vi "Patch of Unflatten Json String.vi"(7 "VCluster":variant, 8 "error in (no error)":errorcluster, 11 "Variant in":variant) -> (0 "error out":errorcluster, 3 "Variant out":variant)   [LabVIEW 2019, in "lv-apt-json-file.lvlib"]
uses:
  lv-apt-json-file.lvlib
  <vilib>/Utility/Data Type/NI_Data Type.lvlib
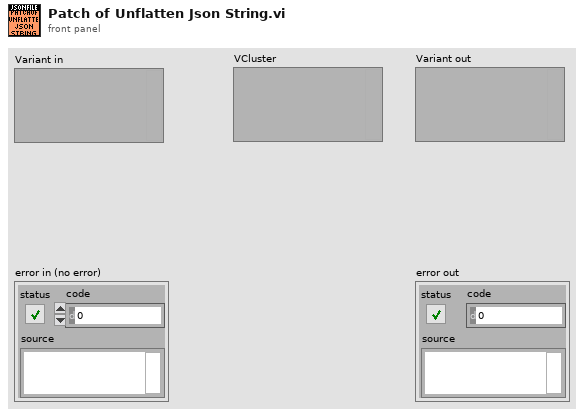
[diagram p1: front panel]
types:
  T1 = typedef "NI_Data Type.lvlib/Data Type.ctl" = enum8{"Invalid Type", "Void", "I8", "I16", "I32", "I64", "U8", "U16", "U32", "U64", "Single Float", "Double Float", "Extended Float", "Single Complex", "Double Complex", "Extended Complex", "Enum U8", "Enum U16", "Enum U32", "Enum U64", "Single Float With Unit", "Double Float With Unit", "Extended Float With Unit", "Single Complex with Unit", "Double Complex with Unit", "Extended Complex with Unit", "Boolean", "String", "Path", "Picture", "Tag", "Array", "Cluster", "Variant", "LV Variant", "Waveform", "Timestamp", "Digital Waveform", "Digital Data", "ExpressData", "Refnum", "External Data", "VI", "Poly VI", "LabVIEW Class Instance", "Fixed Point", "Set Collection", "Map Collection"}
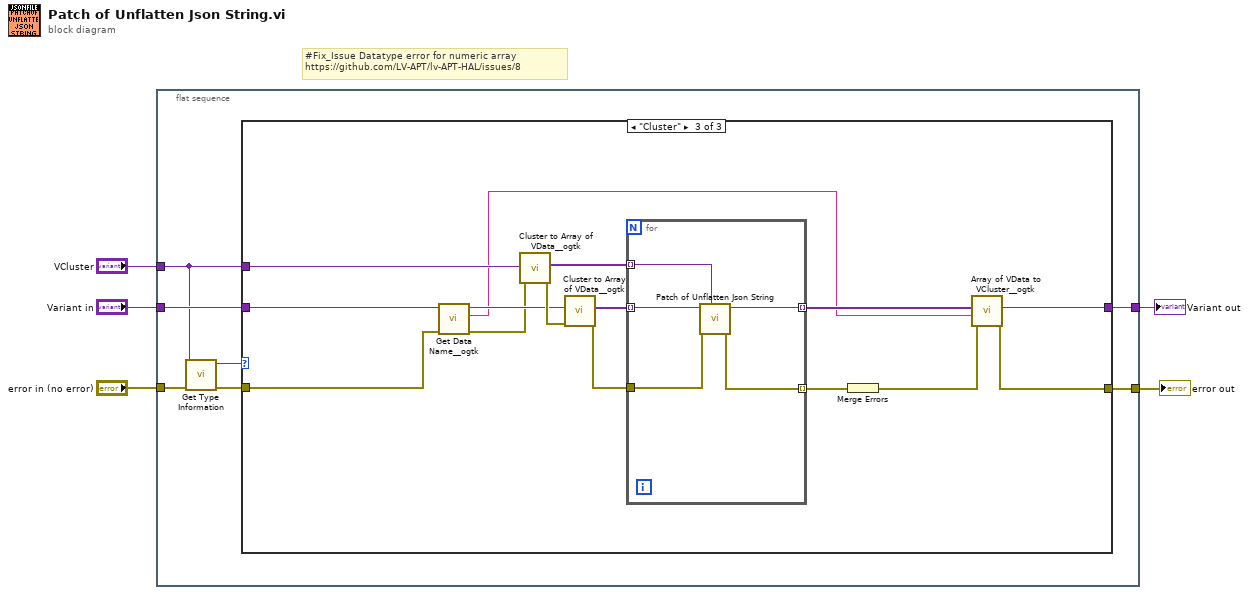
[diagram p0: block diagram]
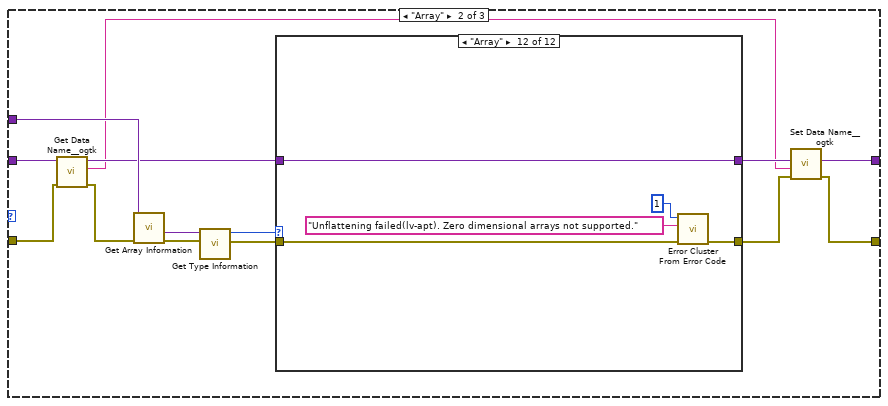
[diagram p3: hidden frame]
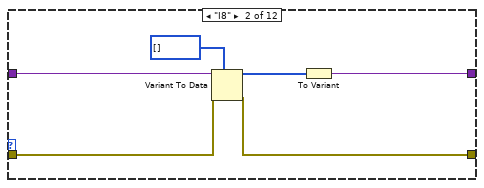
[diagram p5: hidden frame]
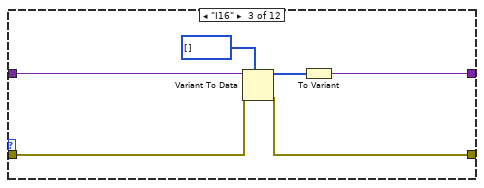
[diagram p6: hidden frame]
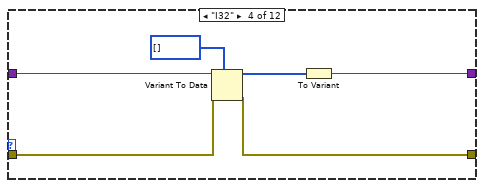
[diagram p7: hidden frame]
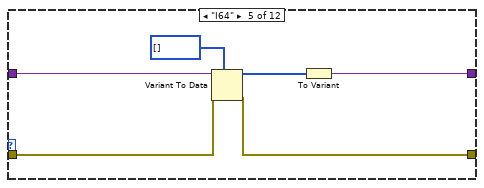
[diagram p8: hidden frame]
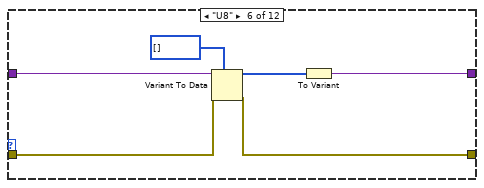
[diagram p9: hidden frame]
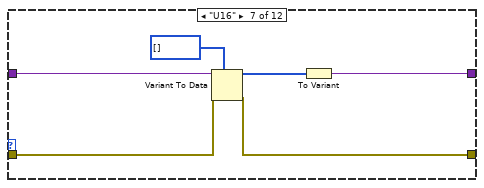
[diagram p10: hidden frame]
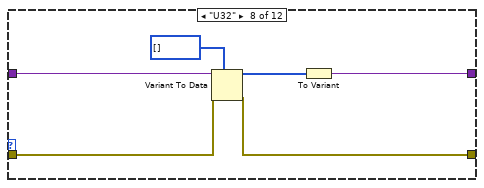
[diagram p11: hidden frame]
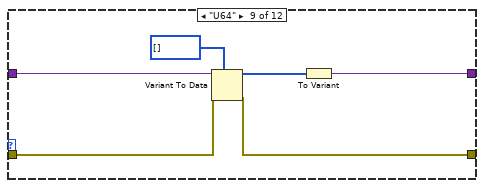
[diagram p12: hidden frame]
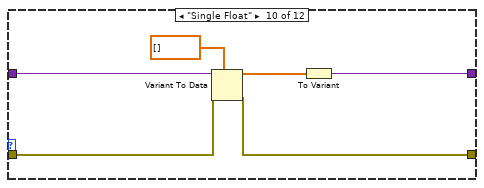
[diagram p13: hidden frame]
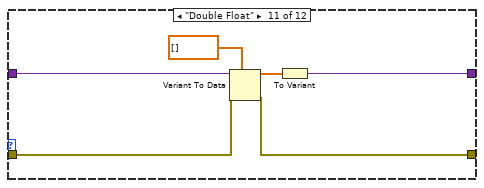
[diagram p14: hidden frame]
diagram:
  # "#Fix_Issue Datatype error for numeric array\nhttps://github.com/LV-APT/lv-APT-HAL/issues/8"
  n1 = flat-sequence {
    tunnel: [w12] -> w1
    tunnel: "Variant in" -> [w11]
    tunnel: "error in (no error)" -> [w9]
    tunnel: [w7] -> w4
    tunnel: "VCluster" -> [w6]
    frame #0 {
      n2 = call <vilib>:"Get Type Information.vi"("error in (no error)"=w9, "variant"=w6) -> ("error out"=w8:errorcluster, "type"=w10:T1)  [unwired: 5 in, 3 out]
      n3 = case shown="\"Cluster\"" w10 {
        tunnel: w11 -> [w14 w24 w110]
        tunnel: [w14 w20 w103] -> w12
        tunnel: w8 -> [w13 w19 w96]
        tunnel: [w13 w15 w100] -> w7
        tunnel: w6 -> [_ w22 w109]
        frame "Invalid Type", Default {
        }
        frame "Array" {
          n4 = call <userlib>:"Get Data Name__ogtk.vi"("error in (no error)"=w19, "Data"=w24) -> ("error out"=w18:errorcluster, "Data Name"=w17:string, "Data dup"=w21:variant)  [unwired: 7 in]
          n5 = call <vilib>:"Get Array Information.vi"("error in (no error)"=w18, "variant"=w22) -> ("error out"=w27:errorcluster, "array element data type"=w28:variant)  [unwired: 6 in, 2 out]
          n6 = call <vilib>:"Get Type Information.vi"("error in (no error)"=w27, "variant"=w28) -> ("error out"=w25:errorcluster, "type"=w26:T1)  [unwired: 5 in, 3 out]
          n7 = case shown="\"Array\"" w26 {
            tunnel: w25 -> [w29 w35 w41 w47 w53 w59 w65 w71 w77 w83 w89 w93]
            tunnel: [w29 w34 w40 w46 w52 w58 w64 w70 w76 w82 w88 w92] -> w16
            tunnel: w21 -> [w30 w36 w42 w48 w54 w60 w66 w72 w78 w84 w90 w91]
            tunnel: [w30 w31 w37 w43 w49 w55 w61 w67 w73 w79 w85 w91] -> w23
            frame Default {
            }
            frame "I8" {
              n8 = Variant To Data(error in=w35, type=i8[] [], Variant=w36) -> (data=w32:i8[], error out=w34:errorcluster)
              n9 = To Variant(anything=w32) -> (Variant=w31:variant)
            }
            frame "I16" {
              n10 = Variant To Data(error in=w41, type=i16[] [], Variant=w42) -> (data=w38:i16[], error out=w40:errorcluster)
              n11 = To Variant(anything=w38) -> (Variant=w37:variant)
            }
            frame "I32" {
              n12 = Variant To Data(error in=w47, type=i32[] [], Variant=w48) -> (data=w44:i32[], error out=w46:errorcluster)
              n13 = To Variant(anything=w44) -> (Variant=w43:variant)
            }
            frame "I64" {
              n14 = Variant To Data(error in=w53, type=i64[] [], Variant=w54) -> (data=w50:i64[], error out=w52:errorcluster)
              n15 = To Variant(anything=w50) -> (Variant=w49:variant)
            }
            frame "U8" {
              n16 = Variant To Data(error in=w59, type=u8[] [], Variant=w60) -> (data=w56:u8[], error out=w58:errorcluster)
              n17 = To Variant(anything=w56) -> (Variant=w55:variant)
            }
            frame "U16" {
              n18 = Variant To Data(error in=w65, type=u16[] [], Variant=w66) -> (data=w62:u16[], error out=w64:errorcluster)
              n19 = To Variant(anything=w62) -> (Variant=w61:variant)
            }
            frame "U32" {
              n20 = Variant To Data(error in=w71, type=u32[] [], Variant=w72) -> (data=w68:u32[], error out=w70:errorcluster)
              n21 = To Variant(anything=w68) -> (Variant=w67:variant)
            }
            frame "U64" {
              n22 = Variant To Data(error in=w77, type=u64[] [], Variant=w78) -> (data=w74:u64[], error out=w76:errorcluster)
              n23 = To Variant(anything=w74) -> (Variant=w73:variant)
            }
            frame "Single Float" {
              n24 = Variant To Data(error in=w83, type=sgl[] [], Variant=w84) -> (data=w80:sgl[], error out=w82:errorcluster)
              n25 = To Variant(anything=w80) -> (Variant=w79:variant)
            }
            frame "Double Float" {
              n26 = Variant To Data(error in=w89, type=dbl[] [], Variant=w90) -> (data=w86:dbl[], error out=w88:errorcluster)
              n27 = To Variant(anything=w86) -> (Variant=w85:variant)
            }
            frame "Array" {
              n28 = call <vilib>:"Error Cluster From Error Code.vi"("error in (no error)"=w93, "error message (\"\")"="Unflattening failed(lv-apt). Zero dimensional arrays not supported." ("error message (\"\")"), "error code (0)"=1) -> ("error out"=w92:errorcluster)  [unwired: 6 in]
            }
          }
          n29 = call <userlib>:"Set Data Name__ogtk.vi"("error in (no error)"=w16, "Data Name"=w17, "Data"=w23) -> ("error out"=w15:errorcluster, "Renamed Data"=w20:variant)  [unwired: 7 in]
        }
        frame "Cluster" {
          n30 = call <userlib>:"Get Data Name__ogtk.vi"("error in (no error)"=w96, "Data"=w110) -> ("error out"=w97:errorcluster, "Data Name"=w98:string, "Data dup"=w99:variant)  [unwired: 7 in]
          n31 = call <userlib>:"Cluster to Array of VData__ogtk.vi"("error in (no error)"=w97, "Cluster"=w109) -> ("error out"=w108:errorcluster, "Array of VData"=w106:variant[])  [unwired: 8 in]
          n32 = call <userlib>:"Cluster to Array of VData__ogtk.vi"("error in (no error)"=w108, "Cluster"=w99) -> ("error out"=w105:errorcluster, "Array of VData"=w107:variant[])  [unwired: 8 in]
          n33 = for {
            tunnel: w107 -> [w115] mode=indexing
            tunnel: w106 -> [w114] mode=indexing
            tunnel: w105 -> [w113]
            tunnel: [w112] -> w104 mode=indexing
            tunnel: [w111] -> w102 mode=indexing
            n34 = call "Patch of Unflatten Json String.vi"("VCluster"=w114, "error in (no error)"=w113, "Variant in"=w115) -> ("error out"=w111:errorcluster, "Variant out"=w112:variant)  [unwired: 7 in]
          }
          n35 = Merge Errors(w102) -> (w101:errorcluster)
          n36 = call <userlib>:"Array of VData to VCluster__ogtk.vi"("error in (no error)"=w101, "Cluster Name"=w98, "Array"=w104) -> ("error out"=w100:errorcluster, "VCluster"=w103:variant)  [unwired: 7 in]
        }
      }
    }
  }
  "error out" <- w4
  "Variant out" <- w1
